vi "Field Replace System Value In Array.vi"(3 "System Field to Replace (Serial Number)":T1=enum."Serial_Number", 4 "Field Value Replacement Data (\"\")":string, 5 "Fields Array In":T2[](array[typedef])) -> (2 "Fields Array Out":T2[](array[typedef]))   [LabVIEW 2011]
uses:
  typedefs/Field Record.ctl
  typedefs/Field DataTypes.ctl
  typedefs/Field NextItem.ctl
  typedefs/Field System Fields.ctl
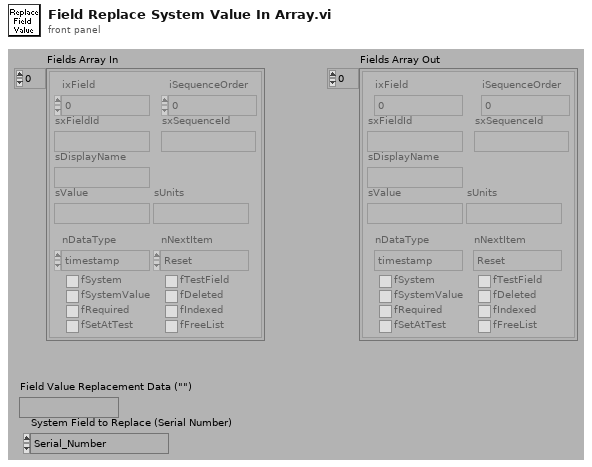
[diagram p1: front panel]
types:
  T1 = typedef "Field System Fields.ctl" = enum32{"Company", "End_Timestamp", "Model_Number", "Operator", "Serial_Number", "Start_Timestamp", "Step_Number", "Step_Tag", "Test_Run", "Test_Sequence", "Test_Station", "Test_Station_Name", "Test_Status", "Test_Type", "Test_Version", "Spartan_Version_Created", "Spartan_Version_Current"}
  T2 = typedef "Field Record.ctl" = cluster{"ixField":i32, "iSequenceOrder":i32, "sxFieldId":string, "sxSequenceId":string, "sDisplayName":string, "sValue":string, "sUnits":string, "nDataType":T3, "nNextItem":T4, "fSystem":bool, "fSystemValue":bool, "fRequired":bool, "fSetAtTest":bool, "fTestField":bool, "fDeleted":bool, "fIndexed":bool, "fFreeList":bool}
  T3 = typedef "Field DataTypes.ctl" = enum32{"text", "numeric", "list", "timestamp", "boolean"}
  T4 = typedef "Field NextItem.ctl" = enum32{"Reset", "Retain", "Auto-Increment"}
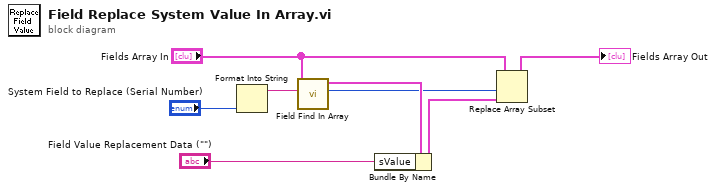
[diagram p0: block diagram]
diagram:
  n1 = Format Into String("System Field to Replace (Serial Number)") -> (resulting string=w2:string)  [unwired: 3 in, 1 out]
  n2 = call "Field Find In Array.vi"("FieldID or Display Name(\"\")"=w2, "Field Array"="Fields Array In") -> ("Index"=w4:i32, "Field"=w6:T2)  [unwired: 1 in, 7 out]
  n3 = Bundle By Name(cluster=w6, "sValue"="Field Value Replacement Data (\"\")") -> (w7:T2)
  n4 = Replace Array Subset(array="Fields Array In", new element=w7, index=w4) -> (→"Fields Array Out":T2[])
